vi "CheckVersion.vi"(10 "Array":T1[](array[typedef]), 11 "Cluster in":T2) -> (2 "Checkbox":bool, 3 "Cluster out":T1)   [LabVIEW 2019, in "ByteLVDevEnv.lvlib"]
uses:
  ByteLVDevEnv.lvlib
  TypeDefs/AllLibraries.ctl
  TypeDefs/LibraryVersions.ctl
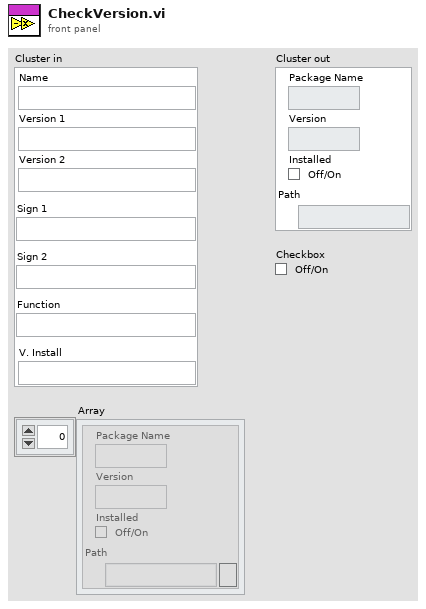
[diagram p1: front panel]
types:
  T1 = typedef "AllLibraries.ctl" = cluster{"Package Name":string, "Version":string, "Installed":bool, "Path":path}
  T2 = typedef "LibraryVersions.ctl" = cluster{"Name":string, "Version 1 ":string, "Version 2":string, "Sign 1":string, "Sign 2":string, "Function":string, "V. Install":string}
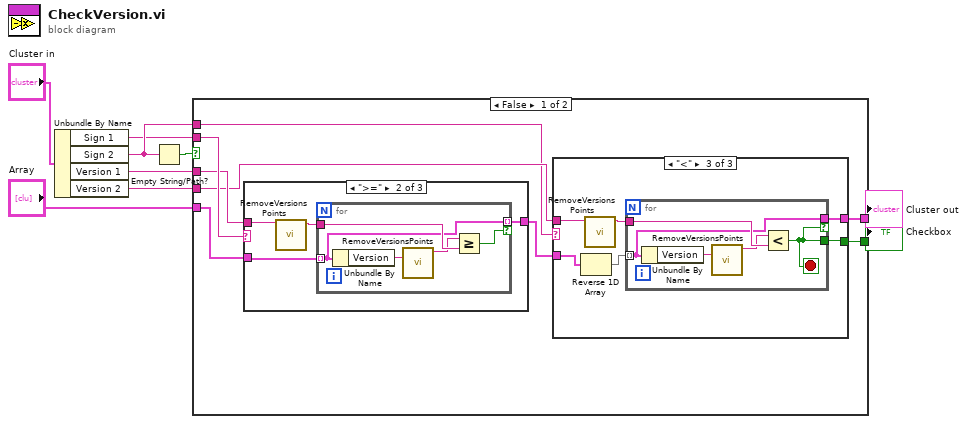
[diagram p0: block diagram]
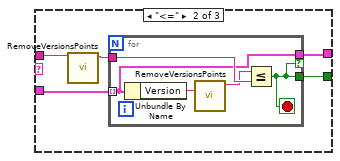
[diagram p3: hidden frame]
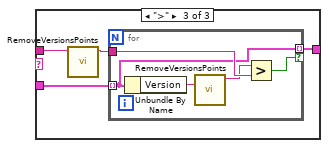
[diagram p5: hidden frame]
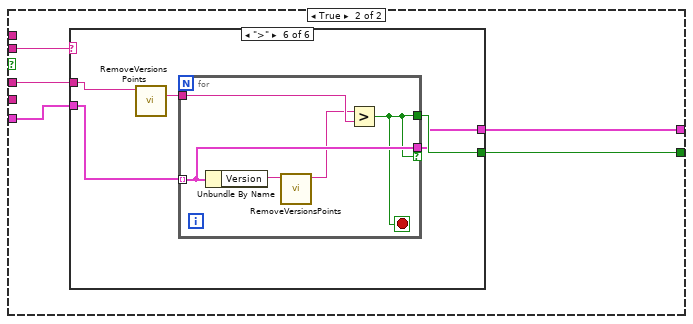
[diagram p6: hidden frame]
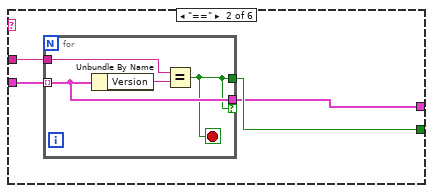
[diagram p8: hidden frame]
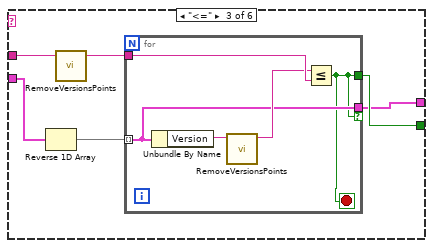
[diagram p9: hidden frame]
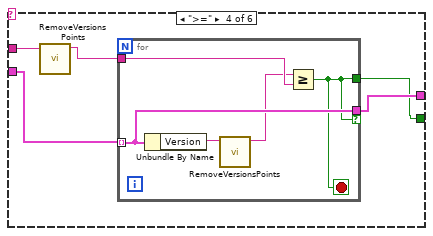
[diagram p10: hidden frame]
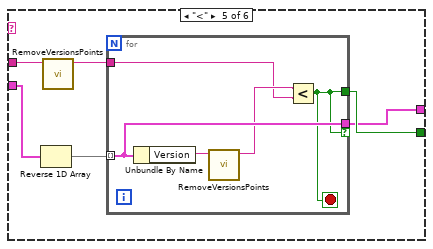
[diagram p11: hidden frame]
diagram:
  n1 = Unbundle By Name("Cluster in") -> ("Sign 1"=w6:string, "Sign 2"=w9:string, "Version 1"=w7:string, "Version 2"=w8:string)
  n2 = Empty String/Path?(string/path=w9) -> (empty?=w5:bool)
  n3 = case shown="False" w5 {
    tunnel: w6 -> [w17 w61]
    tunnel: "Array" -> [w15 w60]
    tunnel: w7 -> [w16 w59]
    tunnel: w8 -> [w14 _]
    tunnel: w9 -> [w12 _]
    tunnel: [w11 w57] -> w4
    tunnel: [w10 w58] -> w3
    frame False {
      n4 = case shown="\">=\"" w17 {
        tunnel: w16 -> [_ w41 w50]
        tunnel: w15 -> [_ w40 w49]
        tunnel: [_ w39 w48] -> w13
        frame Default {
        }
        frame ">=" {
          n5 = call "RemoveVersionsPoints.vi"("Version 1"=w41) -> ("result string"=w42:string)  [unwired: 10 in]
          n6 = for {
            tunnel: w42 -> [w47]
            tunnel: [w43] -> w39 mode=indexing if=w44
            tunnel: w40 -> [w43] mode=indexing
            n7 = Unbundle By Name(w43) -> ("Version"=w45:string)
            n8 = call "RemoveVersionsPoints.vi"("Version 1"=w45) -> ("result string"=w46:string)  [unwired: 10 in]
            n9 = Greater Or Equal?(x=w46, y=w47) -> (x >= y?=w44:bool)
          }
        }
        frame ">" {
          n10 = call "RemoveVersionsPoints.vi"("Version 1"=w50) -> ("result string"=w51:string)  [unwired: 10 in]
          n11 = for {
            tunnel: w51 -> [w56]
            tunnel: [w52] -> w48 mode=indexing if=w53
            tunnel: w49 -> [w52] mode=indexing
            n12 = Unbundle By Name(w52) -> ("Version"=w54:string)
            n13 = call "RemoveVersionsPoints.vi"("Version 1"=w54) -> ("result string"=w55:string)  [unwired: 10 in]
            n14 = Greater?(x=w55, y=w56) -> (0:w53:bool)
          }
        }
      }
      n15 = case shown="\"<\"" w12 {
        tunnel: w14 -> [_ w21 w32]
        tunnel: w13 -> [_ w20 w31]
        tunnel: [_ w19 w29] -> w11
        tunnel: [_ w18 w28] -> w10
        frame Default {
        }
        frame "<=" {
          n16 = call "RemoveVersionsPoints.vi"("Version 1"=w21) -> ("result string"=w22:string)  [unwired: 10 in]
          n17 = for {
            tunnel: w22 -> [w27]
            tunnel: [w24] -> w19 if=w23
            tunnel: w20 -> [w24] mode=indexing
            tunnel: [w23] -> w18
            stop <- w23 stop-if-true
            n18 = Unbundle By Name(w24) -> ("Version"=w25:string)
            n19 = call "RemoveVersionsPoints.vi"("Version 1"=w25) -> ("result string"=w26:string)  [unwired: 10 in]
            n20 = Less Or Equal?(x=w26, y=w27) -> (x <= y?=w23:bool)
          }
        }
        frame "<" {
          n21 = Reverse 1D Array(array=w31) -> (reversed array=w30:T1[])
          n22 = call "RemoveVersionsPoints.vi"("Version 1"=w32) -> ("result string"=w33:string)  [unwired: 10 in]
          n23 = for {
            tunnel: w33 -> [w38]
            tunnel: [w35] -> w29 if=w34
            tunnel: w30 -> [w35] mode=indexing
            tunnel: [w34] -> w28
            stop <- w34 stop-if-true
            n24 = Unbundle By Name(w35) -> ("Version"=w36:string)
            n25 = call "RemoveVersionsPoints.vi"("Version 1"=w36) -> ("result string"=w37:string)  [unwired: 10 in]
            n26 = Less?(x=w37, y=w38) -> (x < y?=w34:bool)
          }
        }
      }
    }
    frame True {
      n27 = case shown="\">\"" w61 {
        tunnel: w60 -> [_ w65 w74 w83 w94 w105]
        tunnel: w59 -> [_ w64 w75 w85 w95 w104]
        tunnel: [_ w63 w71 w81 w92 w103] -> w58
        tunnel: [_ w62 w70 w82 w91 w102] -> w57
        frame Default {
        }
        frame "==" {
          n28 = for {
            tunnel: w65 -> [w67] mode=indexing
            tunnel: w64 -> [w68]
            tunnel: [w67] -> w62 if=w66
            tunnel: [w66] -> w63
            stop <- w66 stop-if-true
            n29 = Unbundle By Name(w67) -> ("Version"=w69:string)
            n30 = Equal?(x=w68, y=w69) -> (x = y?=w66:bool)
          }
        }
        frame "<=" {
          n31 = Reverse 1D Array(array=w74) -> (reversed array=w73:T1[])
          n32 = call "RemoveVersionsPoints.vi"("Version 1"=w75) -> ("result string"=w72:string)  [unwired: 10 in]
          n33 = for {
            tunnel: w73 -> [w77] mode=indexing
            tunnel: w72 -> [w80]
            tunnel: [w77] -> w70 if=w76
            tunnel: [w76] -> w71
            stop <- w76 stop-if-true
            n34 = Unbundle By Name(w77) -> ("Version"=w79:string)
            n35 = call "RemoveVersionsPoints.vi"("Version 1"=w79) -> ("result string"=w78:string)  [unwired: 10 in]
            n36 = Less Or Equal?(x=w78, y=w80) -> (x <= y?=w76:bool)
          }
        }
        frame ">=" {
          n37 = call "RemoveVersionsPoints.vi"("Version 1"=w85) -> ("result string"=w84:string)  [unwired: 10 in]
          n38 = for {
            tunnel: w83 -> [w89] mode=indexing
            tunnel: w84 -> [w87]
            tunnel: [w89] -> w82 if=w88
            tunnel: [w88] -> w81
            stop <- w88 stop-if-true
            n39 = Unbundle By Name(w89) -> ("Version"=w90:string)
            n40 = call "RemoveVersionsPoints.vi"("Version 1"=w90) -> ("result string"=w86:string)  [unwired: 10 in]
            n41 = Greater Or Equal?(x=w86, y=w87) -> (x >= y?=w88:bool)
          }
        }
        frame "<" {
          n42 = Reverse 1D Array(array=w94) -> (reversed array=w93:T1[])
          n43 = call "RemoveVersionsPoints.vi"("Version 1"=w95) -> ("result string"=w96:string)  [unwired: 10 in]
          n44 = for {
            tunnel: w93 -> [w100] mode=indexing
            tunnel: w96 -> [w98]
            tunnel: [w100] -> w91 if=w97
            tunnel: [w97] -> w92
            stop <- w97 stop-if-true
            n45 = Unbundle By Name(w100) -> ("Version"=w101:string)
            n46 = call "RemoveVersionsPoints.vi"("Version 1"=w101) -> ("result string"=w99:string)  [unwired: 10 in]
            n47 = Less?(x=w99, y=w98) -> (x < y?=w97:bool)
          }
        }
        frame ">" {
          n48 = call "RemoveVersionsPoints.vi"("Version 1"=w104) -> ("result string"=w106:string)  [unwired: 10 in]
          n49 = for {
            tunnel: w105 -> [w110] mode=indexing
            tunnel: w106 -> [w108]
            tunnel: [w110] -> w102 if=w109
            tunnel: [w109] -> w103
            stop <- w109 stop-if-true
            n50 = Unbundle By Name(w110) -> ("Version"=w111:string)
            n51 = call "RemoveVersionsPoints.vi"("Version 1"=w111) -> ("result string"=w107:string)  [unwired: 10 in]
            n52 = Greater?(x=w107, y=w108) -> (0:w109:bool)
          }
        }
      }
    }
  }
  "Cluster out" <- w4
  "Checkbox" <- w3
